vi "TxDataDeal.vi"(8 "error in (no error)":errorcluster caption="错误输入（无错误）", 9 "TxdataQ":dbl[](array[numeric]), 10 "TxdataI":dbl[](array[numeric]), 11 "Path":path) -> (0 "error out":errorcluster caption="错误输出", 3 "dataIQ":u16[](array[numeric]))   [LabVIEW 2015]
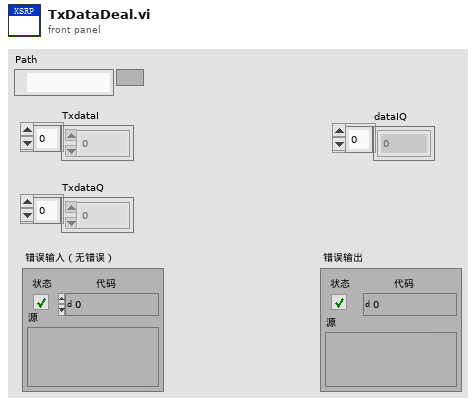
[diagram p1: front panel]
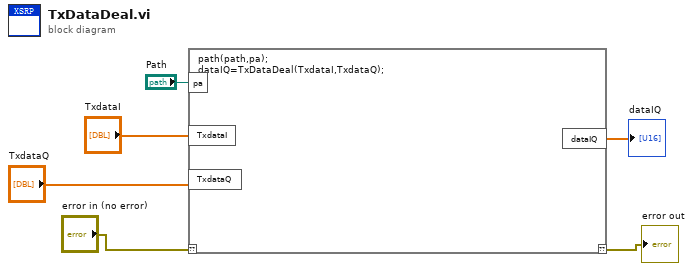
[diagram p0: block diagram]
diagram:
  n1 = script code="path(path,pa);\ndataIQ=TxDataDeal(TxdataI,TxdataQ);"("??"="error in (no error)", "pa"="Path", "TxdataI"="TxdataI", "TxdataQ"="TxdataQ") -> ("??"=→"error out":errorcluster, "dataIQ"=→"dataIQ":dbl[])
